vi "FGSD Calibration tool ver 1.1.2.vi"() -> ()   [LabVIEW 2018]
uses:
  <vilib>/Utility/NIReport.llb/NI_report.lvclass
  <vilib>/Utility/NIReport.llb/Excel/NI_Excel.lvclass
  <vilib>/Utility/NIReport.llb/Report Type.ctl
  <vilib>/DAQmx/read.llb/DAQmx Read (Analog Wfm 1Chan NSamp).vi
  <vilib>/Utility/NIReport.llb/Append Text Table to Report (wrap).vi
  <vilib>/DAQmx/create/channels.llb/DAQmx Create Channel (AI-Voltage-Basic).vi
  <vilib>/DAQmx/configure/timing.llb/DAQmx Timing (Sample Clock).vi
  <vilib>/DAQmx/miscellaneous.llb/DAQmx Fill In Error Info.vi
  <vilib>/Utility/NIReport.llb/Append Numeric Table to Report (wrap).vi
  <vilib>/Utility/NIReport.llb/NI_ReportGenerationCore.lvlib
  <resource>/objmgr/daqmx.rc
panel:
  in  "physical channels 2":tag="Dev1/ao0"
  in  "physical channels":tag="Dev1/ai0"
  in  "Run Next":bool
  in  "Continue":bool
  in  "Unit":enum16{"oz.in", "lbf-ft.", "lbf-in.", "N-m"}(ring)=enum."lbf-in."
  in  "Sensor ID:":tag="BLRTSX 5447375"
  in  "samples per channel":i32=4000
  in  "rate":dbl=500.0 format="%#_13g"
  in  "milliseconds to wait":u32=1000
  out "Cycles":i32=10
  out "Average":dbl[](array[numeric])=[4.1684834279029745]
  out "Template":refnum<class "NI_report.lvclass">
  out "Upper Limit":dbl=4.24
  out "Lower Limit":dbl=3.76
  out "output array":dbl[][](array[numeric])=[[4.141082528801645, 4.21072648068419, 4.134232304026312, 4.192459214616638, 4.1445076411893105], [4.095414363632762, 4.191317510487416, 4.16620001964453, 4.198167735262748, 4.21072648068419]]
  in  "stop":bool
  out "Torque":dbl=4.141082528801645 format="%0.2f"
  out "Waveform Graph 2":waveform(dbl)(graph)={"t0"=timestamp(3675336889.4377584 s since 1904-01-01), "dt"=0.002, "Y"=array[4000 elements], "attributes"=variant("NI_ChannelName"=variant(string "Dev6/ai0"), "NI_UnitDescription"=variant(string "Nm"))}
  out "Torque:":dbl=4.0
  in  "Humidity(%):":string="40"
  in  "Temp(F):":string="75"
  in  "FG Serial Number:":string="0211932-0056"
  in  "User Name:":string="Kyle Watts"
  in  "FG Model:":string(combo)="FG-40i"
  in  "Cal Dir:":string(combo)="CW"
  # "FGSD Calibration Tester ver1.1.2"
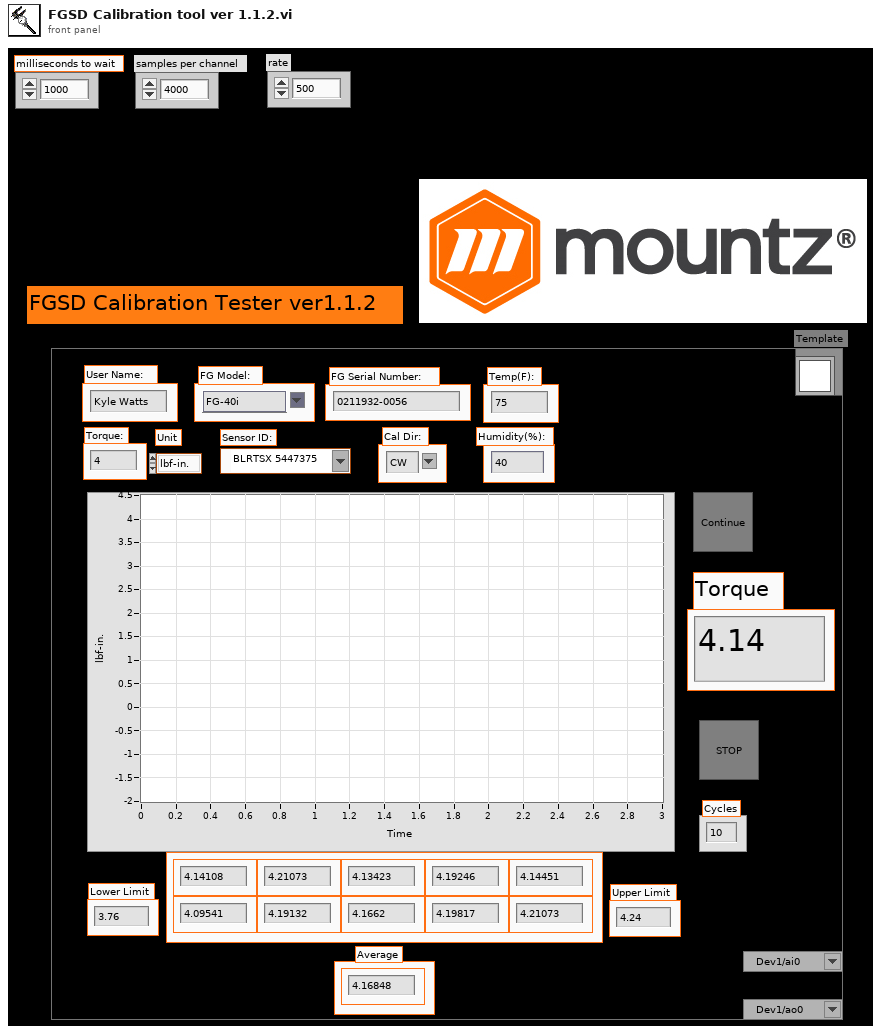
[diagram p1: front panel]
types:
  T1 = enum16{"Initialize ", "Set Torque", "Read Torque"}
  T2 = enum16{"Initialize ", "Set Torque", "Read Torque", "Save data"}
  T3 = cluster{"position (excel)":cluster{"row":i32, "column":i32}, "name (excel)":string, "bookmark (word)":string}
  T4 = cluster{"Charset (-1)":i16, "Weight (-1)":i16, "Name":string, "Size":string}
  T5 = typedef "NI_ReportGenerationCore.lvlib/Report Type.ctl" = enum16{"HTML", "Word", "Excel"}
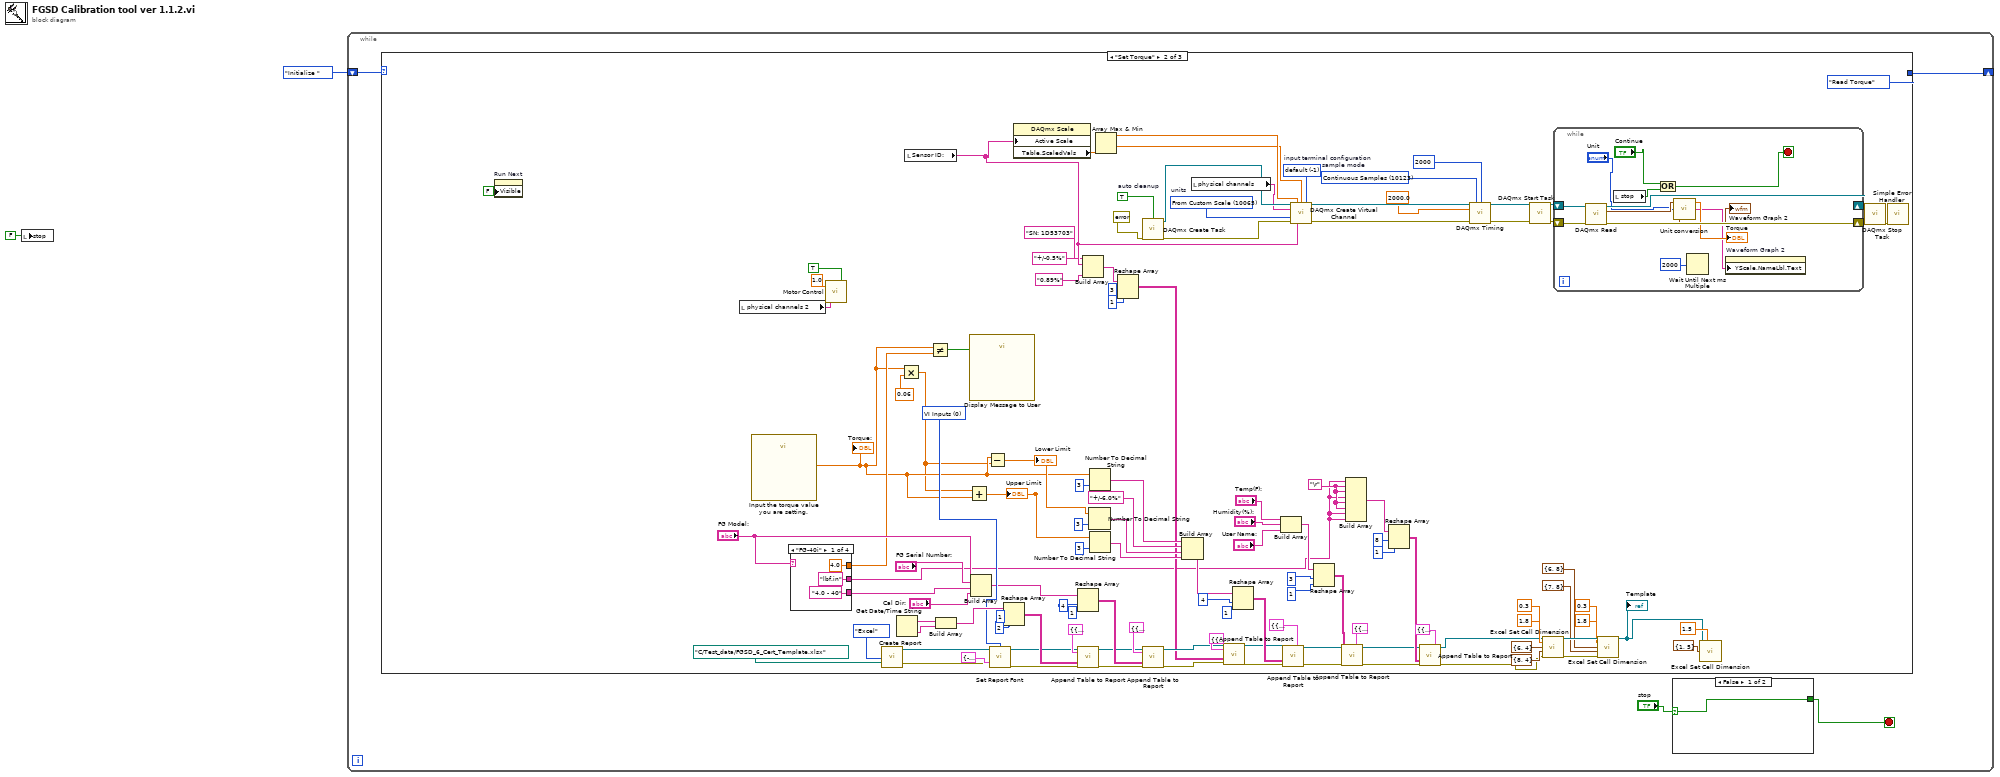
[diagram p0: block diagram]
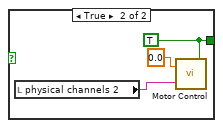
[diagram p2: hidden frame]
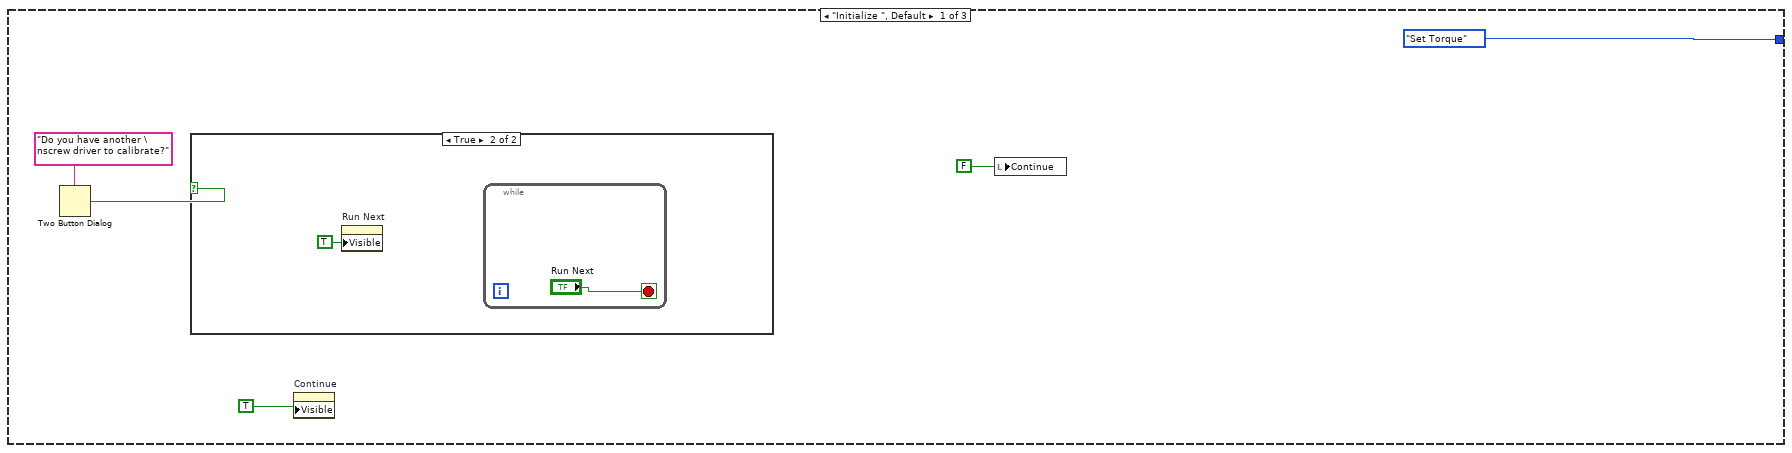
[diagram p3: hidden frame]
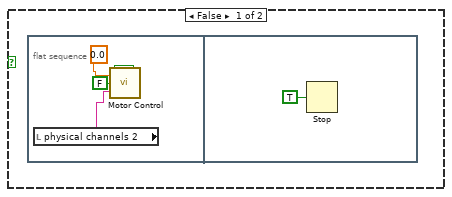
[diagram p4: hidden frame]
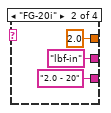
[diagram p5: hidden frame]
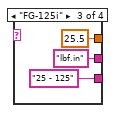
[diagram p6: hidden frame]
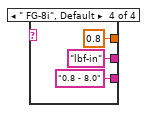
[diagram p7: hidden frame]
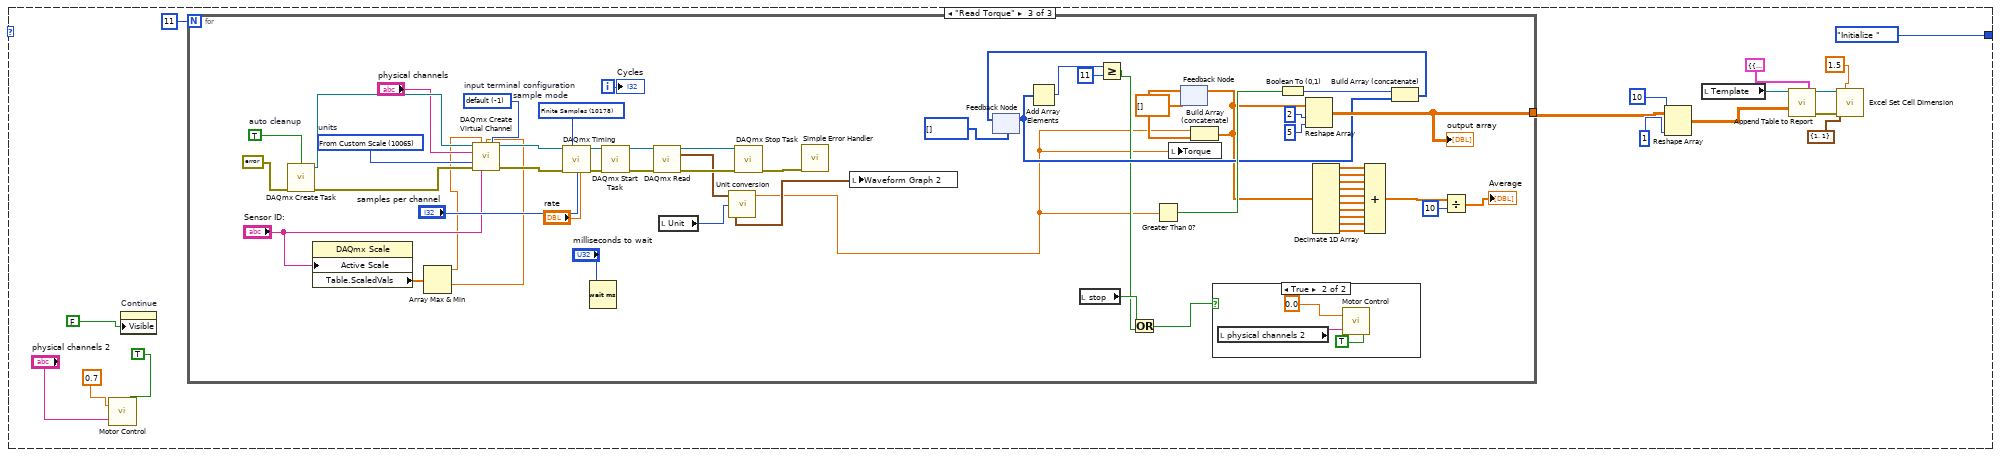
[diagram p8: hidden frame]
diagram:
  n1 = local write "stop"(FALSE ("stop")) -> ()
  n2 = while {
    shift-right: [w5] -> _
    shift-left: T1."Initialize " -> [w6]
    stop <- w3 stop-if-true
    n3 = case shown="\"Set Torque\"" w6 {
      tunnel: [T2."Set Torque" T2."Read Torque" T2."Initialize "] -> w5
      frame "Initialize ", Default {
        n4 = Two Button Dialog(message="Do you have another \nscrew driver to calibrate?") -> (T button?=w12:bool)  [unwired: 2 in]
        n5 = case shown="True" w12 {
          frame False {
            n6 = flat-sequence {
              frame #0 {
                n7 = local read "physical channels 2"() -> (w16:tag)
                n8 = call "Motor Control.vi"("Run"=FALSE, "physical channels"=w16, "Speed"=0.0) -> ()
              }
              frame #1 {
                n9 = Stop(stop? (T)=TRUE) -> ()
              }
            }
          }
          frame True {
            n10 = property on="Run Next" class="Bool"("Visible"=TRUE) -> ()  [unwired: 2 in, 2 out]
            n11 = while {
              stop <- "Run Next" stop-if-true
            }
          }
        }
        n12 = property on="Continue" class="Bool (strict)"("Visible"=TRUE) -> ()  [unwired: 2 in, 2 out]
        n13 = local write "Continue"(FALSE ("Continue")) -> ()
      }
      frame "Set Torque" {
        w32 = "\r"
        w86 = 10123 items=["Finite Samples"=10178, "Continuous Samples"=10123, "Hardware Timed Single Point"=12522]  # sample mode
        w84 = -1 items=["default"=-1, "RSE"=10083, "NRSE"=10078, "Differential"=10106, "Pseudodifferential"=12529]  # input terminal configuration
        w83 = 10065 items=["Volts"=10348, "From Custom Scale"=10065]  # units
        w80 = TRUE  # auto cleanup
        w125 = u16 0 items=["VI Inputs", "Font Dialog Box"] ("font settings source (VI Inputs)")
        n14 = property on="Run Next" class="Bool"("Visible"=FALSE) -> ()  [unwired: 2 in, 2 out]
        n15 = local read "physical channels 2"() -> (w42:tag)
        n16 = call "Input the torque value you are setting."() -> ("Torque"=w23:dbl)  [unwired: 17 in, 2 out]
        "Torque:" <- w23
        n17 = case shown="\"FG-40i\"" "FG Model:" {
          tunnel: ["4.0 - 40" "2.0 - 20" "25 - 125" "0.8 - 8.0"] -> w66
          tunnel: [4.0 2.0 25.5 0.8] -> w96
          tunnel: ["lbf.in" "lbf-in" "lbf.in" "lbf-in"] -> w31
          frame "FG-40i" {
          }
          frame "FG-20i" {
          }
          frame "FG-125i" {
          }
          frame " FG-8i", Default {
          }
        }
        n18 = call "Motor Control.vi"("Run"=TRUE, "physical channels"=w42, "Speed"=1.0) -> ()
        n19 = call <vilib>:"Create Report.vi"("report type"=Report_Type."Excel", "template (empty)"=path "C:/Test_data/FGSD_6_Cert_Template.xlsx") -> ("report out"=w124:refnum<class "NI_report.lvclass">, "error out"=w123:errorcluster)  [unwired: 12 in]
        n20 = Get Date/Time String() -> (date string=w130:string, time string=w131:string)  [unwired: 3 in]
        n21 = Multiply(x=w23, y=0.06) -> (x*y=w22:dbl)
        n22 = local read "Sensor ID:"() -> (w57:tag)
        n23 = Not Equal?(x=w23, y=w96) -> (x != y?=w95:bool)
        n24 = Build Array(w130, w131) -> (w134:string[])
        n25 = Add(x=w22, y=w23) -> (x+y=w58:dbl)
        "Upper Limit" <- w58
        n26 = call "Display Message to User"("Enable"=w95) -> ()  [unwired: 9 in, 2 out]
        n27 = Build Array("FG Model:", "FG Serial Number:", w66, "Cal Dir:") -> (w108:string[])
        n28 = Subtract(x=w23, y=w22) -> (x-y=w59:dbl)
        "Lower Limit" <- w59
        n29 = call-dynamic "Set Report Font.vi"("report in"=w124, "font settings source (VI Inputs)"=w125, "font settings"=T4 {"Charset (-1)"=-1, "Weight (-1)"=-1, "Name"="Calibri", "Size"=" 14"}, "error in (no error)"=w123) -> ("report out"=w121:refnum<class "NI_report.lvclass">, "error out"=w122:errorcluster)  [unwired: 9 in, 1 out]
        n30 = Reshape Array(w134, 1 ("dimension size"), 2 ("dimension size")) -> (w133:string[][])
        n31 = property class="DAQmx Scale"("Active Scale"=w57) -> ("Table.ScaledVals"=w71:dbl[])  [unwired: 2 in, 2 out]
        n32 = Reshape Array(w108, 4 ("dimension size"), 1 ("dimension size")) -> (w107:string[][])
        n33 = call-poly <vilib>:"Append Table to Report.vi"("report in"=w121, "MS Office parameters"=T3 {"position (excel)"={"row"=11, "column"=5}, "name (excel)"="", "bookmark (word)"=""}, "text data"=w133, "error in (no error)"=w122) -> ("report out"=w105:refnum<class "NI_report.lvclass">, "error out"=w104:errorcluster)  [unwired: 8 in, 2 out]
        n34 = Build Array("SN: 1D53703", w57, "+/-0.5%", "0.89%") -> (w54:string[])
        n35 = Number To Decimal String(number=w59, width (-)=i16 3) -> (decimal integer string=w61:string)
        n36 = Number To Decimal String(number=w23, width (-)=i16 3) -> (decimal integer string=w63:string)
        n37 = Number To Decimal String(number=w58, width (-)=i16 3) -> (decimal integer string=w60:string)
        n38 = Array Max & Min(array=w71) -> (max value=w70:dbl, min value=w69:dbl)  [unwired: 2 out]
        n39 = Reshape Array(w54, 3 ("dimension size"), 1 ("dimension size")) -> (w51:string[][])
        n40 = call <vilib>:"DAQmx Create Task.vi"("auto cleanup"=w80, "error in"=errorcluster {"status"=FALSE, "code"=0, "source"=""}) -> ("task out"=w81:refnum<k21>, "error out"=w79:errorcluster)  [unwired: 12 in]
        n41 = call-poly <vilib>:"Append Table to Report.vi"("report in"=w105, "MS Office parameters"=T3 {"position (excel)"={"row"=11, "column"=1}, "name (excel)"="", "bookmark (word)"=""}, "text data"=w107, "error in (no error)"=w104) -> ("report out"=w127:refnum<class "NI_report.lvclass">, "error out"=w128:errorcluster)  [unwired: 8 in, 2 out]
        n42 = Build Array(w63, "+/-6.0%", w61, w60) -> (w103:string[])
        n43 = local read "physical channels"() -> (w41:tag)
        n44 = call-poly <vilib>:"Append Table to Report.vi"("report in"=w127, "MS Office parameters"=T3 {"position (excel)"={"row"=16, "column"=5}, "name (excel)"="", "bookmark (word)"=""}, "text data"=w51, "error in (no error)"=w128) -> ("report out"=w46:refnum<class "NI_report.lvclass">, "error out"=w64:errorcluster)  [unwired: 8 in, 2 out]
        n45 = Reshape Array(w103, 4 ("dimension size"), 1 ("dimension size")) -> (w100:string[][])
        n46 = Build Array("Temp(F):", "Humidity(%):", "User Name:") -> (w97:string[])
        n47 = call-poly <vilib>:"Append Table to Report.vi"("report in"=w46, "MS Office parameters"=T3 {"position (excel)"={"row"=16, "column"=1}, "name (excel)"="", "bookmark (word)"=""}, "text data"=w100, "error in (no error)"=w64) -> ("report out"=w44:refnum<class "NI_report.lvclass">, "error out"=w45:errorcluster)  [unwired: 8 in, 2 out]
        n48 = call-poly <vilib>:"DAQmx Create Virtual Channel.vi"("task in"=w81, "maximum value"=w70, "minimum value"=w69, "input terminal configuration"=w84, "physical channels"=w41, "units"=w83, "error in"=w79, "custom scale name"=w57) -> ("task out"=w85:refnum<k21>, "error out"=w82:errorcluster)  [unwired: 6 in]
        n49 = Reshape Array(w97, 3 ("dimension size"), 1 ("dimension size")) -> (w47:string[][])
        n50 = call-poly <vilib>:"Append Table to Report.vi"("report in"=w44, "MS Office parameters"=T3 {"position (excel)"={"row"=12, "column"=5}, "name (excel)"="", "bookmark (word)"=""}, "text data"=w47, "error in (no error)"=w45) -> ("report out"=w30:refnum<class "NI_report.lvclass">, "error out"=w29:errorcluster)  [unwired: 8 in, 2 out]
        n51 = Build Array(w31, w32, w32, w31, w32, w32, w31, w31) -> (w35:string[])
        n52 = Reshape Array(w35, 8 ("dimension size"), 1 ("dimension size")) -> (w34:string[][])
        n53 = call-poly <vilib>:"Append Table to Report.vi"("report in"=w30, "MS Office parameters"=T3 {"position (excel)"={"row"=13, "column"=2}, "name (excel)"="", "bookmark (word)"=""}, "text data"=w34, "error in (no error)"=w29) -> ("report out"=w28:refnum<class "NI_report.lvclass">, "error out"=w27:errorcluster)  [unwired: 8 in, 2 out]
        n54 = call-poly <vilib>:"DAQmx Timing.vi"("task/channels in"=w85, "sample mode"=w86, "samples per channel"=2000, "rate"=2000.0, "error in"=w82) -> ("task out"=w88:refnum<k21>, "error out"=w78:errorcluster)  [unwired: 9 in]
        n55 = call <vilib>:"DAQmx Start Task.vi"("task/channels in"=w88, "error in"=w78) -> ("task out"=w90:refnum<k21>, "error out"=w89:errorcluster)  [unwired: 12 in]
        n56 = call <vilib>:"Excel Set Cell Dimension.vi"("report in"=w28, "width (-1)"=1.8, "height (-1)"=0.3, "start (-1, -1)"=cluster{"row":i32, "column":i32} {"row"=6, "column"=4}, "end (-1, -1)"=cluster{"row":i32, "column":i32} {"row"=8, "column"=4}, "error in (no error)"=w27) -> ("report out"=w116:refnum<class "NI_report.lvclass">, "error out"=w115:errorcluster)  [unwired: 8 in]
        n57 = while {
          shift-right: [w151] -> w76
          shift-left: w90 -> [w153]
          shift-right: [w150] -> w75
          shift-left: w89 -> [w152]
          stop <- w148 stop-if-true
          n58 = call-poly <vilib>:"DAQmx Read.vi"("task/channels in"=w153, "error in"=w152) -> ("task out"=w151:refnum<k21>, "data"=w146:waveform(dbl), "error out"=w150:errorcluster)  [unwired: 11 in]
          n59 = local read "stop"() -> (w149:bool)
          n60 = Or(x="Continue", y=w149) -> (x .or. y?=w148:bool)
          n61 = call "Unit conversion.vi"("Convert to"="Unit", "data in"=w146) -> ("Unit"=w142:string, "Torque"=→"Torque":dbl, "waveform out"=→"Waveform Graph 2":waveform(dbl))  [unwired: 1 in]
          n62 = Wait Until Next ms Multiple(millisecond multiple=u32 2000) -> ()  [unwired: 1 out]
          n63 = property on="Waveform Graph 2" class="WFGraph (strict)"("YScale.NameLbl.Text"=w142) -> ()  [unwired: 2 in, 2 out]
        }
        n64 = call <vilib>:"Excel Set Cell Dimension.vi"("report in"=w116, "width (-1)"=1.8, "height (-1)"=0.3, "start (-1, -1)"=cluster{"row":i32, "column":i32} {"row"=6, "column"=8}, "end (-1, -1)"=cluster{"row":i32, "column":i32} {"row"=7, "column"=8}, "error in (no error)"=w115) -> ("report out"=w38:refnum<class "NI_report.lvclass">)  [unwired: 8 in, 1 out]
        "Template" <- w38
        n65 = call <vilib>:"Excel Set Cell Dimension.vi"("report in"=w38, "width (-1)"=1.5, "start (-1, -1)"=cluster{"row":i32, "column":i32} {"row"=1, "column"=5} ("end (-1, -1)")) -> ()  [unwired: 11 in, 2 out]
        n66 = call <vilib>:"DAQmx Stop Task.vi"("task/channels in"=w76, "error in"=w75) -> ("error out"=w74:errorcluster)  [unwired: 12 in, 1 out]
        n67 = call <vilib>:"Simple Error Handler.vi"("error in (no error)"=w74) -> ()  [unwired: 4 in, 5 out]
      }
      frame "Read Torque" {
        n68 = call "Motor Control.vi"("Run"=TRUE, "physical channels"="physical channels 2", "Speed"=0.7) -> ()
        n69 = property on="Continue" class="Bool (strict)"("Visible"=FALSE) -> ()  [unwired: 2 in, 2 out]
        n70 = for {
          N: 11 -> [_]
          tunnel: [w239] -> w178
          i -> [w213]
          w198 = 10178 items=["Finite Samples"=10178, "Continuous Samples"=10123, "Hardware Timed Single Point"=12522]  # sample mode
          w195 = -1 items=["default"=-1, "RSE"=10083, "NRSE"=10078, "Differential"=10106, "Pseudodifferential"=12529]  # input terminal configuration
          w193 = 10065 items=["Volts"=10348, "From Custom Scale"=10065]  # units
          w192 = TRUE  # auto cleanup
          n71 = call <vilib>:"DAQmx Create Task.vi"("auto cleanup"=w192, "error in"=errorcluster {"status"=FALSE, "code"=0, "source"=""}) -> ("task out"=w204:refnum<k21>, "error out"=w203:errorcluster)  [unwired: 12 in]
          n72 = property class="DAQmx Scale"("Active Scale"="Sensor ID:") -> ("Table.ScaledVals"=w188:dbl[])  [unwired: 2 in, 2 out]
          n73 = Array Max & Min(array=w188) -> (max value=w187:dbl, min value=w186:dbl)  [unwired: 2 out]
          n74 = call-poly <vilib>:"DAQmx Create Virtual Channel.vi"("task in"=w204, "maximum value"=w187, "minimum value"=w186, "input terminal configuration"=w195, "physical channels"="physical channels", "units"=w193, "error in"=w203, "custom scale name"="Sensor ID:") -> ("task out"=w206:refnum<k21>, "error out"=w205:errorcluster)  [unwired: 6 in]
          n75 = call-poly <vilib>:"DAQmx Timing.vi"("task/channels in"=w206, "sample mode"=w198, "samples per channel"="samples per channel", "rate"="rate", "error in"=w205) -> ("task out"=w207:refnum<k21>, "error out"=w202:errorcluster)  [unwired: 9 in]
          n76 = Wait (ms)(milliseconds to wait="milliseconds to wait") -> ()  [unwired: 1 out]
          n77 = call <vilib>:"DAQmx Start Task.vi"("task/channels in"=w207, "error in"=w202) -> ("task out"=w209:refnum<k21>, "error out"=w208:errorcluster)  [unwired: 12 in]
          n78 = call-poly <vilib>:"DAQmx Read.vi"("task/channels in"=w209, "error in"=w208) -> ("task out"=w201:refnum<k21>, "data"=w185:waveform(dbl), "error out"=w200:errorcluster)  [unwired: 11 in]
          n79 = local read "Unit"() -> (w182:enum16{"oz.in", "lbf-ft.", "lbf-in.", "N-m"})
          n80 = call "Unit conversion.vi"("Convert to"=w182, "data in"=w185) -> ("Torque"=w183:dbl, "waveform out"=w184:waveform(dbl))  [unwired: 1 in, 1 out]
          n81 = call <vilib>:"DAQmx Stop Task.vi"("task/channels in"=w201, "error in"=w200) -> ("error out"=w199:errorcluster)  [unwired: 12 in, 1 out]
          n82 = call <vilib>:"Simple Error Handler.vi"("error in (no error)"=w199) -> ()  [unwired: 4 in, 5 out]
          n83 = local write "Waveform Graph 2"(w184) -> ()
          n84 = feedback #1(i16[] []) -> (w234:i16[])
          n85 = Add Array Elements(numeric array=w234) -> (sum=w236:i16)
          n86 = local read "stop"() -> (w214:bool)
          n87 = Greater Or Equal?(x=w236, y=i16 11) -> (x >= y?=w190:bool)
          n88 = Or(x=w214, y=w190) -> (x .or. y?=w212:bool)
          n89 = Greater Than 0?(x=w183) -> (x > 0?=w238:bool)
          n90 = local write "Torque"(w183) -> ()
          n91 = feedback #2(dbl[] []) -> (w231:dbl[])
          n92 = Build Array (concatenate)(w183, w231) -> (w227:dbl[])
          n93 = feedback-in #2(w227) -> ()
          n94 = case shown="True" w212 {
            frame False {
            }
            frame True {
              n95 = local read "physical channels 2"() -> (w240:tag)
              n96 = call "Motor Control.vi"("Run"=TRUE, "physical channels"=w240, "Speed"=0.0) -> ()
            }
          }
          n97 = Boolean To (0,1)(Boolean=w238) -> (0, 1=w237:i16)
          n98 = Reshape Array(w227, 2 ("dimension size"), 5 ("dimension size")) -> (w239:dbl[][])
          "output array" <- w239
          n99 = Decimate 1D Array(w227) -> (w226:dbl[], w225:dbl[], w224:dbl[], w223:dbl[], w222:dbl[], w221:dbl[], w220:dbl[], w219:dbl[], w218:dbl[], w217:dbl[])
          n100 = Compound Arithmetic op=ADD(w226, w225, w224, w223, w222, w221, w220, w219, w218, w217) -> (w211:dbl[])
          n101 = Build Array (concatenate)(w237, w234) -> (w235:i16[])
          n102 = feedback-in #1(w235) -> ()
          n103 = Divide(x=w211, y=10) -> (x/y=→"Average":dbl[])
          "Cycles" <- w213
        }
        n104 = Reshape Array(w178, 10 ("dimension size"), 1 ("dimension size")) -> (w177:dbl[][])
        n105 = local read "Template"() -> (w175:refnum<class "NI_report.lvclass">)
        n106 = call-poly <vilib>:"Append Table to Report.vi"("report in"=w175, "MS Office parameters"=T3 {"position (excel)"={"row"=23, "column"=1}, "name (excel)"="", "bookmark (word)"=""}, "numerical data"=w177) -> ("report out"=w169:refnum<class "NI_report.lvclass">, "error out"=w168:errorcluster)  [unwired: 9 in, 2 out]
        n107 = call <vilib>:"Excel Set Cell Dimension.vi"("report in"=w169, "width (-1)"=1.5 ("column width (1)"), "start (-1, -1)"=cluster{"row":i32, "column":i32} {"row"=1, "column"=1}, "error in (no error)"=w168) -> ()  [unwired: 10 in, 2 out]
      }
    }
    n108 = case shown="False" "stop" {
      selector: "stop" -> [w7 _]
      tunnel: [w7 w9] -> w3
      frame False {
      }
      frame True {
        w9 = TRUE ("Run")
        n109 = local read "physical channels 2"() -> (w8:tag)
        n110 = call "Motor Control.vi"("Run"=w9, "physical channels"=w8, "Speed"=0.0) -> ()
      }
    }
  }
